vi "Add.vi"(2 "AngleAdd":refnum<class "Angle.lvclass">, 3 "Angle in":refnum<class "Angle.lvclass">) -> (0 "Output":dbl, 1 "?":refnum<class "Angle.lvclass">)   [LabVIEW 2013, in "Angle.lvclass"]
doc: "Bonnie Ishiguro, Fall 2013\n\nTakes two angles as inputs and returns their sum."
uses:
  Angle.lvclass
  Angle.lvclass/Angle.ctl
panel:
  in  "Angle out":refnum<class "Angle.lvclass">
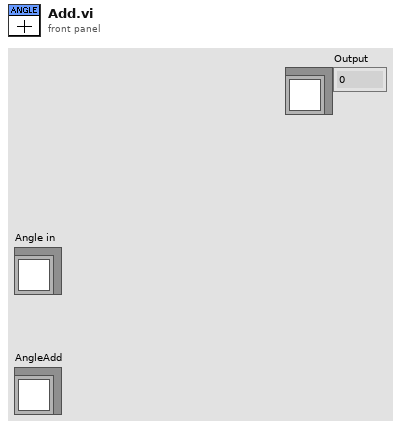
[diagram p1: front panel]
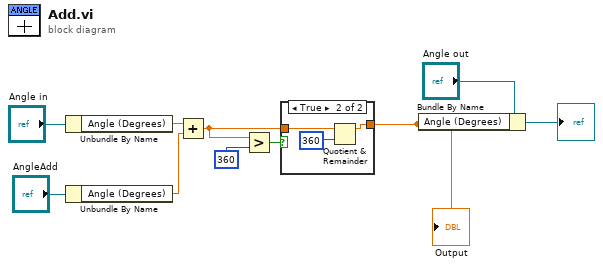
[diagram p0: block diagram]
diagram:
  n1 = Unbundle By Name("Angle in") -> ("Angle (Degrees)"=w9:dbl)
  n2 = Unbundle By Name("AngleAdd") -> ("Angle (Degrees)"=w7:dbl)
  n3 = Add(x=w9, y=w7) -> (x+y=w4:dbl)
  n4 = Greater?(x=w4, y=360) -> (0:w5:bool)
  n5 = case shown="True" w5 {
    tunnel: w4 -> [w11 w13]
    tunnel: [w11 w14] -> w2
    frame False {
    }
    frame True {
      n6 = Quotient & Remainder(x=w13, y=360) -> (x-y*floor(x/y)=w14:dbl)  [unwired: 1 out]
    }
  }
  "Output" <- w2
  n7 = Bundle By Name(cluster="Angle out", "Angle (Degrees)"=w2) -> (→"?":refnum<class "Angle.lvclass">)
